vi "Init SFC.vi"(1 "Algo":string) -> (15 "Control":T1={"queue"=refnum, "error"={"status"=FALSE, "code"=0, "source"=""}, "Step"={"Name"="", "Timeout"=0.0}, "Algorythm"=[{"Name"="Init", "Timeout"=0.0}]})   [LabVIEW 2023, in "SFC.lvlib"]
uses:
  SFC.lvlib
  TypeDef/Step TypeDef.ctl
  TypeDef/Control TypeDef.ctl
panel:
  in  "Step":T2
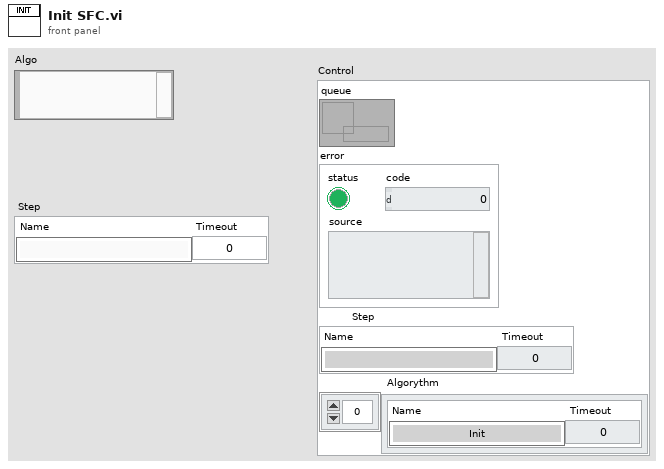
[diagram p1: front panel]
types:
  T1 = typedef "SFC.lvlib/Control TypeDef.ctl" = cluster{"queue":refnum<queue>, "error":errorcluster, "Step":T2, "Algorythm":T2[]}
  T2 = typedef "SFC.lvlib/Step TypeDef.ctl" = cluster{"Name":string, "Timeout":dbl}
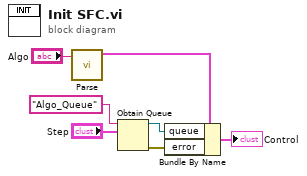
[diagram p0: block diagram]
diagram:
  n1 = call "Parse.vi"("Algo"="Algo") -> ("output cluster"=w1:T1)  [unwired: 10 in]
  n2 = Obtain Queue(name (unnamed)="Algo_Queue", element data type="Step") -> (queue out=w5:refnum<queue>, error out=w4:errorcluster)  [unwired: 3 in, 1 out]
  n3 = Bundle By Name(cluster=w1, "queue"=w5, "error"=w4) -> (→"Control":T1)
